vi "SPC_test_id.vi"(8 "Error In":errorcluster, 10 "Module No":i16 min=0 max=3 step=1, 11 "DLL Path":path) -> (0 "Error Out":errorcluster, 2 "Module No":i16, 3 "DLL Path":path, 4 "Module Name":string)   [LabVIEW 2017]
doc: "The procedure can be used to check whether an SPC module is present and which type of the\nmodule it is. It is a low level procedure that is called also during the initialisation in SPC_init.\nThe procedure returns a module type value of module ‘mod_no’. Possible module type values \nare defined in spcm_def.h file.\nThe x0x and x3x versions are not distinguished by the id but by the EEPROM data and the \nfunction SPC_init. SPC_test_id will return the correct values only if SPC_init has been called.\n/* supported SPC module types - returned value from SPC_test_id */\n#define M_SPC600 600 PCI version of 400\n#define M_SPC630 630 PCI version of 430\n#define M_SPC700 700 PCI version of 500\n#define M_SPC730 730 PCI version of 530\n#define M_SPC130 130 PCI special version of 630\n#define M_SPC830 830 version of 730 with large memory, Fifo mode\n#define M_SPC140 140 130 with large memory, Fifo mode, Scan modes\n#define M_SPC930 930 830 with Camera mode\n#define M_SPC150 150 140 with Fifo mode, Scan modes, Fifo Imaging, Cont. Flow\n#define M_DPC230 230 DPC-230\n#define M_SPC131 131 130 with with extended memory = SPC-130-EM\n#define M_SPC151 151 150N = 150 with faster discriminators and reduced timing wobble\n#define M_SPC160 160 160 - special module for optical tomography\n\ninfo@becker-hickl.com"
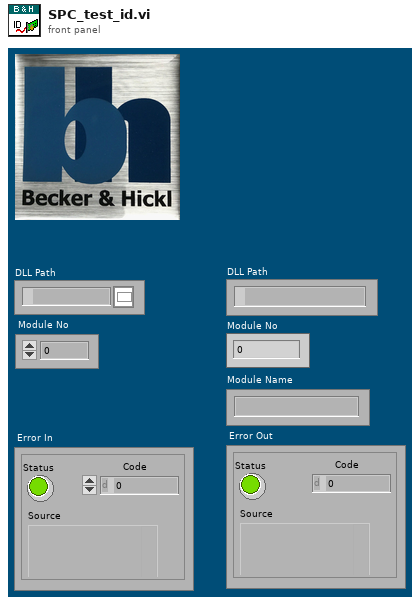
[diagram p1: front panel]
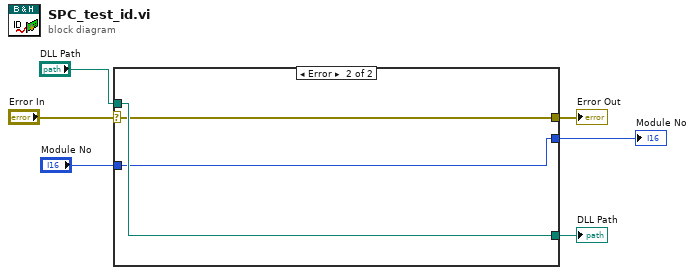
[diagram p0: block diagram]
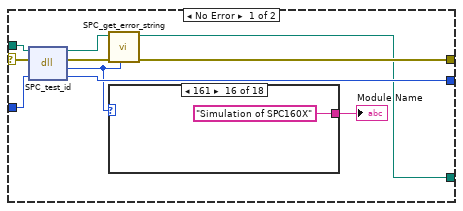
[diagram p2: hidden frame]
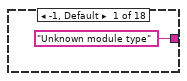
[diagram p3: hidden frame]
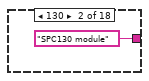
[diagram p4: hidden frame]
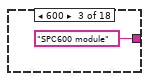
[diagram p5: hidden frame]
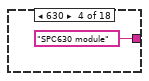
[diagram p6: hidden frame]
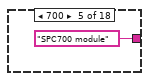
[diagram p7: hidden frame]
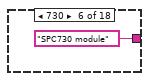
[diagram p8: hidden frame]
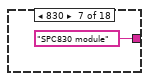
[diagram p9: hidden frame]
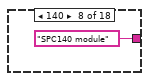
[diagram p10: hidden frame]
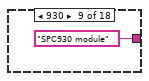
[diagram p11: hidden frame]
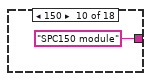
[diagram p12: hidden frame]
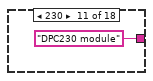
[diagram p13: hidden frame]
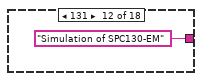
[diagram p14: hidden frame]
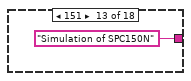
[diagram p15: hidden frame]
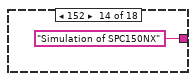
[diagram p16: hidden frame]
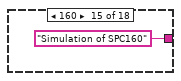
[diagram p17: hidden frame]
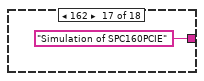
[diagram p18: hidden frame]
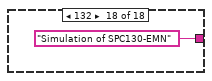
[diagram p19: hidden frame]
diagram:
  n1 = case shown="Error" "Error In" {
    selector: "Error In" -> [w14 w36]
    tunnel: "DLL Path" -> [w15 w37]
    tunnel: [w8 w37] -> w5
    tunnel: [w9 w36] -> w3
    tunnel: "Module No" -> [w13 w35]
    tunnel: [w12 w35] -> w1
    frame No Error {
      n2 = dll-call lib="D:/spcm/lib/lab_view/lv10.0/spcm32.dll" fn="SPC_test_id"(path in=w15, error in=w14, "mod_no"=w13) -> (path out=w7:path, error out=w10:errorcluster, "return type"=w11:i16, "mod_no"=w12:i16)  [unwired: 1 in]
      n3 = call "SPC_get_error_string.vi"("ErrorID"=w11, "Error In"=w10, "DLL Path"=w7) -> ("Error Out"=w9:errorcluster, "DLL Path"=w8:path)  [unwired: 6 in, 1 out]
      n4 = case shown="161" w11 {
        tunnel: ["Unknown module type" "SPC130 module" "SPC600 module" "SPC630 module" "SPC700 module" "SPC730 module" "SPC830 module" "SPC140 module" "SPC930 module" "SPC150 module" "DPC230 module" "Simulation of SPC130-EM" "Simulation of SPC150N" "Simulation of SPC150NX" "Simulation of SPC160" "Simulation of SPC160X" "Simulation of SPC160PCIE" "Simulation of SPC130-EMN"] -> w16
        frame -1, Default {
        }
        frame 130 {
        }
        frame 600 {
        }
        frame 630 {
        }
        frame 700 {
        }
        frame 730 {
        }
        frame 830 {
        }
        frame 140 {
        }
        frame 930 {
        }
        frame 150 {
        }
        frame 230 {
        }
        frame 131 {
        }
        frame 151 {
        }
        frame 152 {
        }
        frame 160 {
        }
        frame 161 {
        }
        frame 162 {
        }
        frame 132 {
        }
      }
      "Module Name" <- w16
    }
    frame Error {
    }
  }
  "DLL Path" <- w5
  "Error Out" <- w3
  "Module No" <- w1
